vi "Simultaneous Start.vi"() -> ()   [LabVIEW 2009]
uses:
  <vilib>/DAQmx/write.llb/DAQmx Write (Analog Wfm 1Chan NSamp).vi
  <vilib>/DAQmx/configure/timing.llb/DAQmx Timing (Sample Clock).vi
  <vilib>/DAQmx/create/channels.llb/DAQmx Create Channel (AO-Voltage-Basic).vi
  <vilib>/DAQmx/configure/trigger.llb/DAQmx Start Trigger (Digital Edge).vi
  <vilib>/DAQmx/create/channels.llb/DAQmx Create Channel (AI-Voltage-Basic).vi
  <vilib>/DAQmx/read.llb/DAQmx Read (Analog 1D DBL 1Chan NSamp).vi
  Program Files/National Instruments/LabVIEW 2009/resource/objmgr/daqmx.rc
  <vilib>/measure/NI_MABase.lvlib
panel:
  out "data":dbl[](graph)
  out "signal out":waveform(dbl)(graph)
  in  "stop":bool
  in  "input rate":dbl=1000.0 format="%0.2f"
  in  "output rate":dbl(slide)=1000.0 scale=100.0..2000.0
  in  "AI channel":tag
  in  "AO channel":tag
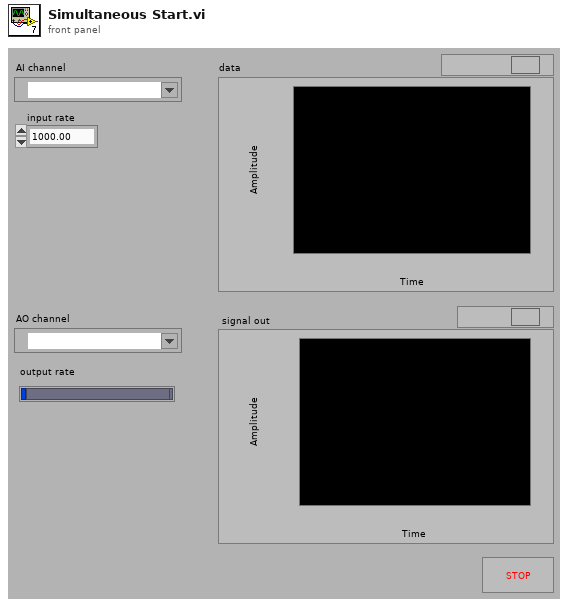
[diagram p1: front panel]
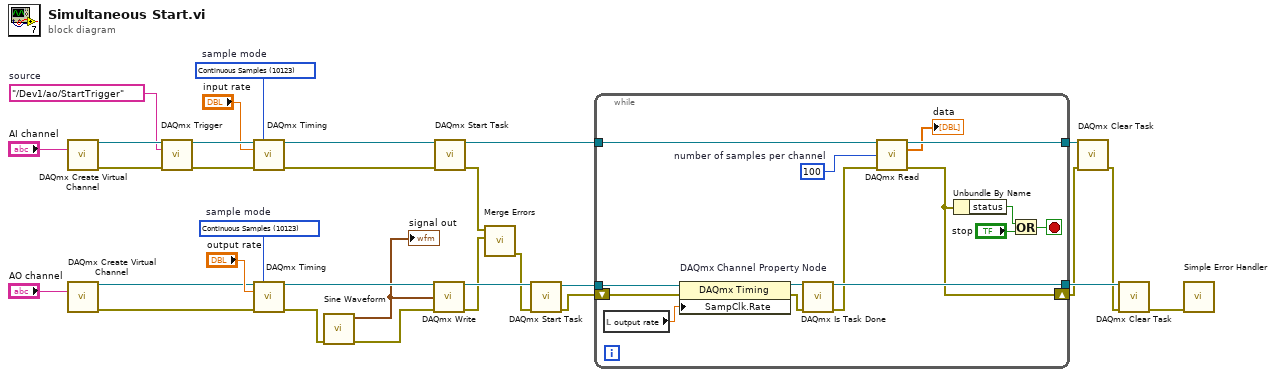
[diagram p0: block diagram]
diagram:
  w8 = tag "/Dev1/ao/StartTrigger"  # source
  w9 = 10123 items=["Finite Samples"=10178, "Continuous Samples"=10123, "Hardware Timed Single Point"=12522]  # sample mode
  w10 = 10123 items=["Finite Samples"=10178, "Continuous Samples"=10123, "Hardware Timed Single Point"=12522]  # sample mode
  n1 = call-poly <vilib>:"DAQmx Create Virtual Channel.vi"("physical channels"="AI channel") -> ("task out"=w27:refnum<k21>, "error out"=w31:errorcluster)  [unwired: 13 in]
  n2 = call-poly <vilib>:"DAQmx Create Virtual Channel.vi"("physical channels"="AO channel") -> ("task out"=w2:refnum<k21>, "error out"=w1:errorcluster)  [unwired: 13 in]
  n3 = call-poly <vilib>:"DAQmx Trigger.vi"("task/channels in"=w27, "source"=w8, "error in"=w31) -> ("task out"=w22:refnum<k21>, "error out"=w20:errorcluster)  [unwired: 11 in]
  n4 = call-poly <vilib>:"DAQmx Timing.vi"("task/channels in"=w22, "sample mode"=w10, "rate"="input rate", "error in"=w20) -> ("task out"=w21:refnum<k21>, "error out"=w3:errorcluster)  [unwired: 10 in]
  n5 = call-poly <vilib>:"DAQmx Timing.vi"("task/channels in"=w2, "sample mode"=w9, "rate"="output rate", "error in"=w1) -> ("task out"=w19:refnum<k21>, "error out"=w13:errorcluster)  [unwired: 10 in]
  n6 = call <vilib>:"Sine Waveform.vi"("error in (no error)"=w13) -> ("error out"=w12:errorcluster, "signal out"=w11:waveform(dbl))  [unwired: 9 in]
  "signal out" <- w11
  n7 = call-poly <vilib>:"DAQmx Write.vi"("task/channels in"=w19, "data"=w11, "error in"=w12) -> ("task out"=w28:refnum<k21>, "error out"=w5:errorcluster)  [unwired: 10 in, 1 out]
  n8 = call <vilib>:"DAQmx Start Task.vi"("task/channels in"=w21, "error in"=w3) -> ("task out"=w26:refnum<k21>, "error out"=w4:errorcluster)  [unwired: 12 in]
  n9 = call <vilib>:"Merge Errors.vi"("error in 2 (no error)"=w5, "error in 1 (no error)"=w4) -> ("error out"=w6:errorcluster)  [unwired: 5 in]
  n10 = call <vilib>:"DAQmx Start Task.vi"("task/channels in"=w28, "error in"=w6) -> ("task out"=w29:refnum<k21>, "error out"=w7:errorcluster)  [unwired: 12 in]
  n11 = while {
    tunnel: [w45] -> w30
    tunnel: w29 -> [w43]
    tunnel: w26 -> [w42]
    tunnel: [w41] -> w25
    shift-right: [w39] -> w16
    shift-left: w7 -> [w33]
    stop <- w36 stop-if-true
    w34 = 100  # number of samples per channel
    n12 = local read "output rate"() -> (w35:dbl)
    n13 = property on="DAQmx Channel Property Node" class="DAQmx Timing"(reference=w43, error in=w33, "SampClk.Rate"=w35) -> (reference out=w44:refnum<k21>, error out=w46:errorcluster)
    n14 = call <vilib>:"DAQmx Is Task Done.vi"("task/channels in"=w44, "error in"=w46) -> ("task out"=w45:refnum<k21>, "error out"=w40:errorcluster)  [unwired: 11 in, 1 out]
    n15 = call-poly <vilib>:"DAQmx Read.vi"("task/channels in"=w42, "number of samples per channel"=w34, "error in"=w40) -> ("task out"=w41:refnum<k21>, "data"=→"data":dbl[], "error out"=w39:errorcluster)  [unwired: 10 in]
    n16 = Unbundle By Name "Unbundle By Name"(w39) -> ("status"=w38:bool)
    n17 = Or(x=w38, y="stop") -> (x .or. y?=w36:bool)
  }
  n18 = call <vilib>:"DAQmx Clear Task.vi"("task in"=w25, "error in"=w16) -> ("error out"=w15:errorcluster)  [unwired: 13 in]
  n19 = call <vilib>:"DAQmx Clear Task.vi"("task in"=w30, "error in"=w15) -> ("error out"=w14:errorcluster)  [unwired: 13 in]
  n20 = call <vilib>:"Simple Error Handler.vi"("error in (no error)"=w14) -> ()  [unwired: 4 in, 5 out]
